vi "whileLoopilesinewave.vi"() -> ()   [LabVIEW 2024]
panel:
  in  "Stop Button 2":bool
  in  "f 2":dbl
  out "Waveform Chart 2":dbl(graph)
  in  "amplitude 2":dbl
  in  "amplitude":dbl
  out "Waveform Chart":dbl(graph)
  out "Concatenated Data Array":dbl[](array[numeric])
  in  "Stop Button":bool
  in  "f":dbl
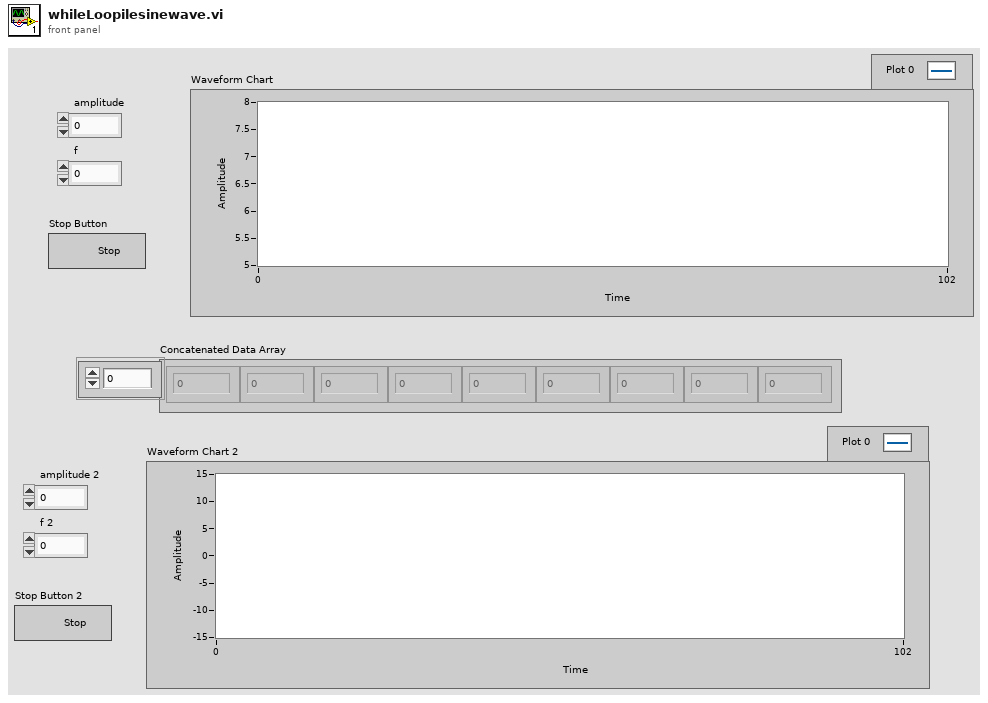
[diagram p1: front panel]
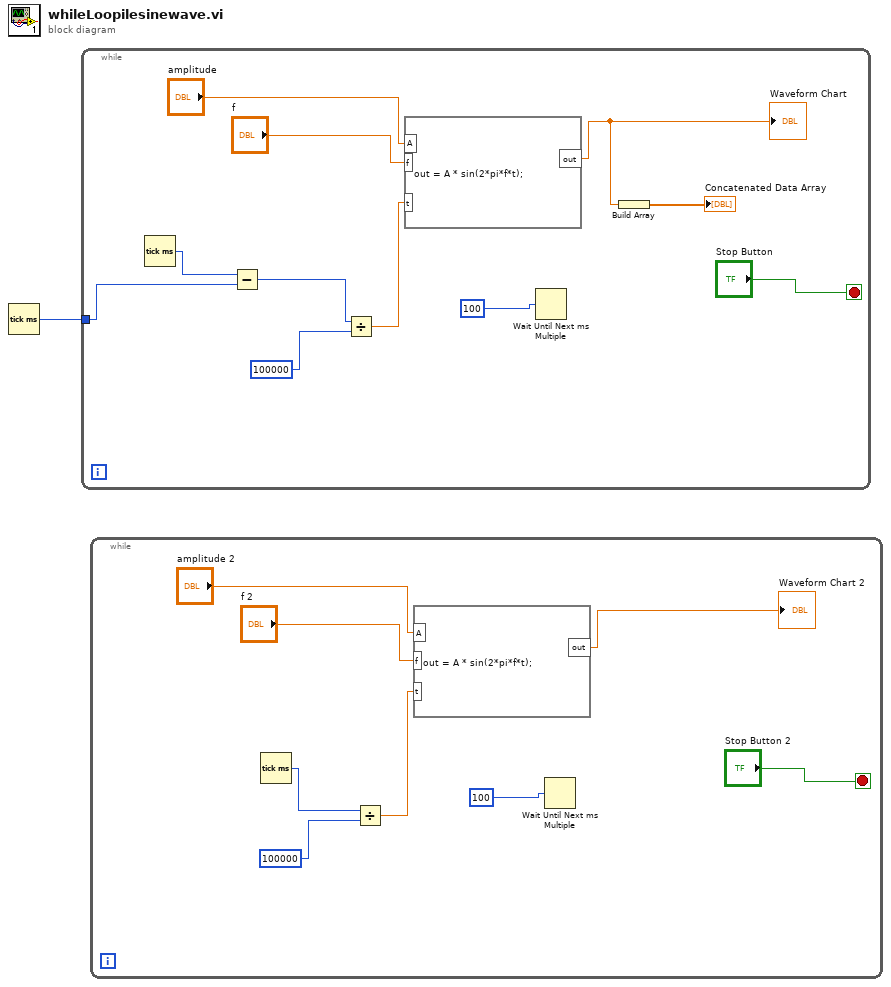
[diagram p0: block diagram]
diagram:
  n1 = Tick Count (ms)() -> (millisecond timer value=w1:u32)
  n2 = while {
    tunnel: w1 -> [w7]
    stop <- "Stop Button" stop-if-true
    n3 = Tick Count (ms)() -> (millisecond timer value=w6:u32)
    n4 = Subtract(x=w6, y=w7) -> (x-y=w2:u32)
    n5 = Divide(x=w2, y=u32 100000) -> (x/y=w4:dbl)
    n6 = formula code="out = A * sin(2*pi*f*t);"("f"="f", "t"=w4, "A"="amplitude") -> ("out"=w9:dbl)
    "Waveform Chart" <- w9
    n7 = Wait Until Next ms Multiple(millisecond multiple=u32 100) -> ()  [unwired: 1 out]
    n8 = Build Array(w9) -> (→"Concatenated Data Array":dbl[])
  }
  n9 = while {
    stop <- "Stop Button 2" stop-if-true
    n10 = Tick Count (ms)() -> (millisecond timer value=w13:u32)
    n11 = Divide(x=w13, y=u32 100000) -> (x/y=w15:dbl)
    n12 = formula code="out = A * sin(2*pi*f*t);"("f"="f 2", "t"=w15, "A"="amplitude 2") -> ("out"=→"Waveform Chart 2":dbl)
    n13 = Wait Until Next ms Multiple(millisecond multiple=u32 100) -> ()  [unwired: 1 out]
  }
